vi "MH_ResizeBuffer.vi"(8 "WinIndex":i32, 9 "Buffindex":i32, 10 "Buffsize":i32, 11 "Tableau":u64[](array[numeric])) -> (0 "NewWinIndex":i32, 1 "NewBuffIndex":i32, 2 "NewBuffsize":i32, 3 "tableau (n rotations)":u64[](array[numeric]), 4 "deltaT Rotate":u32, 5 "Rotation Size":i32)   [LabVIEW 2019]
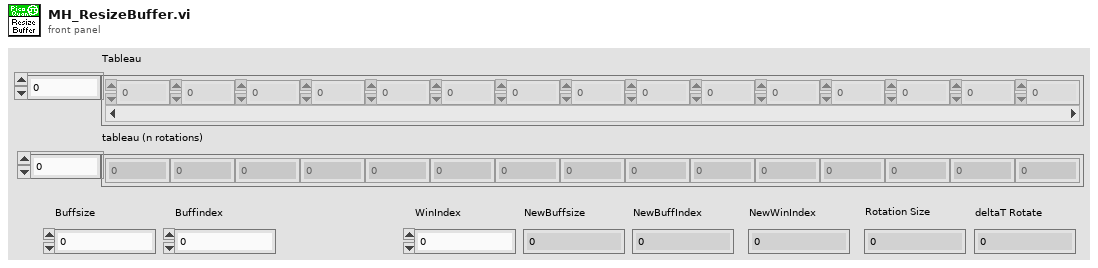
[diagram p1: front panel]
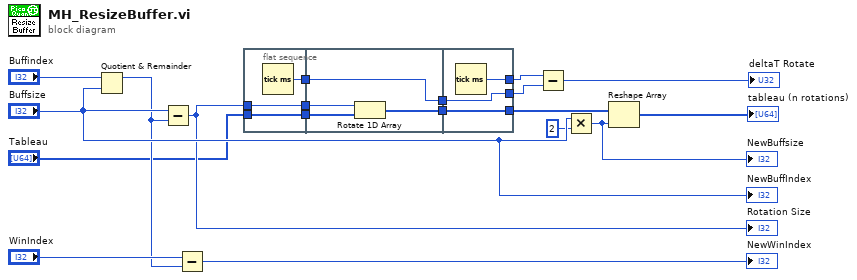
[diagram p0: block diagram]
diagram:
  n1 = Quotient & Remainder(x="Buffindex", y="Buffsize") -> (x-y*floor(x/y)=w14:i32)  [unwired: 1 out]
  n2 = Subtract(x="Buffsize", y=w14) -> (x-y=w16:i32)
  "Rotation Size" <- w16
  n3 = Subtract(x="WinIndex", y=w14) -> (x-y=→"NewWinIndex":i32)
  n4 = flat-sequence {
    tunnel: w16 -> [w21]
    tunnel: "Tableau" -> [w22]
    tunnel: [w22] -> w12
    tunnel: [w21] -> w11
    tunnel: [w20] -> w8
    tunnel: w12 -> [w25]
    tunnel: w11 -> [w24]
    tunnel: [w26] -> w10
    tunnel: [w23] -> w9
    tunnel: w8 -> [w23]
    tunnel: [w29] -> w19
    tunnel: w10 -> [w29]
    tunnel: [w28] -> w6
    tunnel: w9 -> [w28]
    tunnel: [w27] -> w7
    frame #0 {
      n5 = Tick Count (ms)() -> (millisecond timer value=w20:u32)
    }
    frame #1 {
      n6 = Rotate 1D Array(1:w25, 2:w24) -> (0:w26:u64[])
    }
    frame #2 {
      n7 = Tick Count (ms)() -> (millisecond timer value=w27:u32)
    }
  }
  n8 = Subtract(x=w7, y=w6) -> (x-y=→"deltaT Rotate":u32)
  n9 = Multiply(x="Buffsize", y=2) -> (x*y=w2:i32)
  "NewBuffsize" <- w2
  n10 = Reshape Array(w19, w2) -> (→"tableau (n rotations)":u64[])
  "NewBuffIndex" <- "Buffsize"
